vi "ziGetEvent.vi"   [LabVIEW 2009, in "Zurich Instruments LabOne.lvlib"]
doc: "This vi retrieves data from a previous ziPollDataEx.vi call. Use the Path and ziValueType returned by ziPollDataEx.vi to determine, which polymorphic version of ziGetEvent.vi is appropriate.\n\nFor double value and integer value types, no ziGetEvent.vi is required, these two value types are also returned directly by ziPollDataEx.vi."
uses:
  <instrlib>/Zurich Instruments LabOne/Zurich Instruments LabOne.lvlib
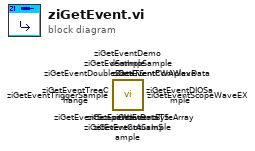
[diagram p0: block diagram]
diagram:
  n1 = call <instrlib>:"ziGetEventIntDataTS.vi"() -> ()  [unwired: 9 in, 3 out]
  n2 = call <instrlib>:"ziGetEventComplexData.vi"() -> ()  [unwired: 9 in, 3 out]
  n3 = call <instrlib>:"ziGetEventTriggerSample.vi"() -> ()  [unwired: 9 in, 3 out]
  n4 = call <instrlib>:"ziGetEventScopeWaveEX.vi"() -> ()  [unwired: 9 in, 3 out]
  n5 = call <instrlib>:"ziGetEventCntSample.vi"() -> ()  [unwired: 9 in, 3 out]
  n6 = call <instrlib>:"ziGetEventImpSample.vi"() -> ()  [unwired: 9 in, 3 out]
  n7 = call <instrlib>:"ziGetEventDoubleDataTS.vi"() -> ()  [unwired: 9 in, 3 out]
  n8 = call <instrlib>:"ziGetEventByteArray.vi"() -> ()  [unwired: 9 in, 3 out]
  n9 = call <instrlib>:"ziGetEventTreeChange.vi"() -> ()  [unwired: 9 in, 3 out]
  n10 = call <instrlib>:"ziGetEventDIOSample.vi"() -> ()  [unwired: 9 in, 3 out]
  n11 = call <instrlib>:"ziGetEventAuxInSample.vi"() -> ()  [unwired: 9 in, 3 out]
  n12 = call <instrlib>:"ziGetEventDemodSample.vi"() -> ()  [unwired: 9 in, 3 out]
  n13 = call <instrlib>:"ziGetEventScopeWave.vi"() -> ()  [unwired: 9 in, 3 out]
  n14 = call <instrlib>:"ziGetEventPWAWave.vi"() -> ()  [unwired: 9 in, 3 out]
